vi "Ping.vi"(11 "IP address":string) -> (0 "cmd Error Out":errorcluster, 3 "Ping Successful?":bool)   [LabVIEW 2014]
panel:
  out "Ping Unsuccessful":bool
  out "Output":string
  out "Last ping":string
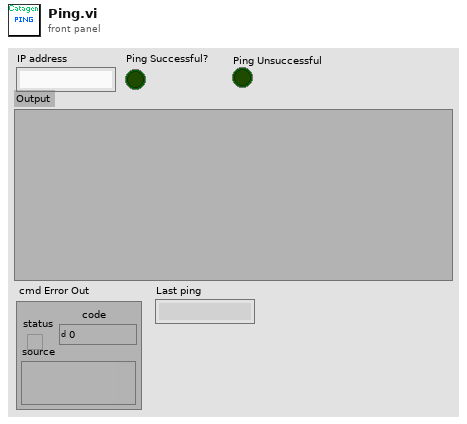
[diagram p1: front panel]
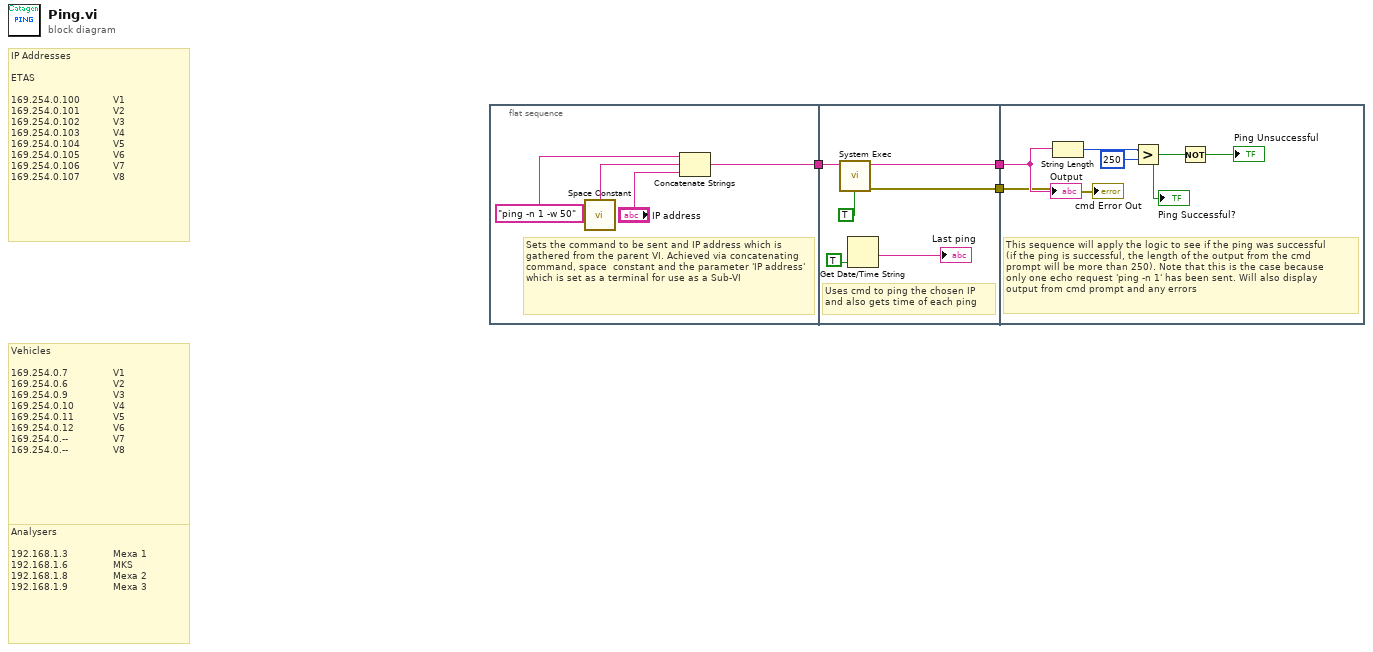
[diagram p0: block diagram]
diagram:
  # "Analysers\n\n192.168.1.3               Mexa 1\n192.168.1.6               MKS\n192.168.1.8               Mexa 2\n192.168.1.9               Mexa 3"
  # "Vehicles\n\n169.254.0.7               V1\n169.254.0.6               V2\n169.254.0.9               V3\n169.254.0.10             V4\n169.254.0.11             V5\n169.254.0.12             V6\n169.254.0.--               V7\n169.254.0.--               V8"
  # "IP Addresses\n\nETAS\n\n169.254.0.100           V1\n169.254.0.101           V2\n169.254.0.102           V3\n169.254.0.103           V4\n169.254.0.104           V5\n169.254.0.105           V6\n169.254.0.106           V7\n169.254.0.107           V8"
  n1 = flat-sequence {
    tunnel: [w7] -> w3
    tunnel: w3 -> [w12]
    tunnel: [w11] -> w2
    tunnel: [w10] -> w1
    tunnel: w2 -> [w16]
    tunnel: w1 -> [w19]
    frame #0 {
      # "Sets the command to be sent and IP address which is gathered from the parent VI. Achieved via concatenating command, space  constant and the parameter 'IP address' which is set as a terminal for use as a Sub-VI"
      n2 = call <vilib>:"Space Constant.vi"() -> ("String"=w5:string)
      n3 = Concatenate Strings("ping -n 1 -w 50", w5, "IP address") -> (w7:string)
    }
    frame #1 {
      # "Uses cmd to ping the chosen IP \nand also gets time of each ping"
      n4 = call <vilib>:"System Exec.vi"("run minimized? (F)"=TRUE, "command line"=w12) -> ("error out"=w11:errorcluster, "standard output"=w10:string)  [unwired: 6 in, 2 out]
      n5 = Get Date/Time String(want seconds? (F)=TRUE) -> (time string=→"Last ping":string)  [unwired: 2 in, 1 out]
    }
    frame #2 {
      # "This sequence will apply the logic to see if the ping was successful \n(if the ping is successful, the length of the output from the cmd \nprompt will be more than 250). Note that this is the case because\nonly one echo request 'ping -n 1' has been sent. Will also display \noutput from cmd prompt and any errors"
      n6 = String Length(string=w19) -> (length=w17:i32)
      n7 = Greater?(x=w17, y=250) -> (0:w15:bool)
      "Ping Successful?" <- w15
      n8 = Not(x=w15) -> (.not. x?=→"Ping Unsuccessful":bool)
      "Output" <- w19
      "cmd Error Out" <- w16
    }
  }
